vi "Add Service.vi"(6 "WebSocket Data Handler":refnum<class "WebSocket Data Handler Msg.lvclass">, 8 "error in (no error)":errorcluster, 9 "Subscriber Enqueuer":refnum<class "Message Enqueuer.lvclass">, 10 "Service Name":string, 11 "WebSocket Server in":refnum<class "WebSocket Server.lvclass">) -> (0 "error out":errorcluster, 3 "WebSocket Server out":refnum<class "WebSocket Server.lvclass">)   [LabVIEW 2016, in "WebSocket Actor.lvlib" / "WebSocket Server.lvclass"]
uses:
  WebSocket Server.lvclass
  C:/Program Files (x86)/National Instruments/LabVIEW 2016/vi.lib/ActorFramework/Actor/Actor.lvclass
  <vilib>/ActorFramework/Message Enqueuer/Message Enqueuer.lvclass
  Abstract Messages/WebSocket Data Handler Msg/WebSocket Data Handler Msg.lvclass
  WebSocket Server.lvclass/WebSocket Server.ctl
  WebSocket Listener Actor/WebSocket Service Actor.lvclass
  WebSocket Listener Actor/WebSocket Service Actor.lvclass/WebSocket Service Actor.ctl
  Abstract Messages/WebSocket Service Enqueuer Msg/WebSocket Service Enqueuer Msg.lvclass/WebSocket Service Enqueuer Msg.ctl
  <vilib>/ActorFramework/Message Enqueuer/Message Enqueuer.lvclass/Message Enqueuer.ctl
  WebSocket Listener Actor/properties/Write Subscriber Enqueuer.vi
  WebSocket Listener Actor/properties/Write WebSocket Data Handler.vi
  <vilib>/ActorFramework/Message Enqueuer/Enqueue.vi
  Abstract Messages/WebSocket Service Enqueuer Msg/WebSocket Service Enqueuer Msg.lvclass
  C:/Program Files (x86)/National Instruments/LabVIEW 2016/vi.lib/ActorFramework/Message/Message.lvclass
  <vilib>/ActorFramework/Message Priority Queue/Priority Enqueue.vi
  <vilib>/ActorFramework/Actor/Actor.lvclass
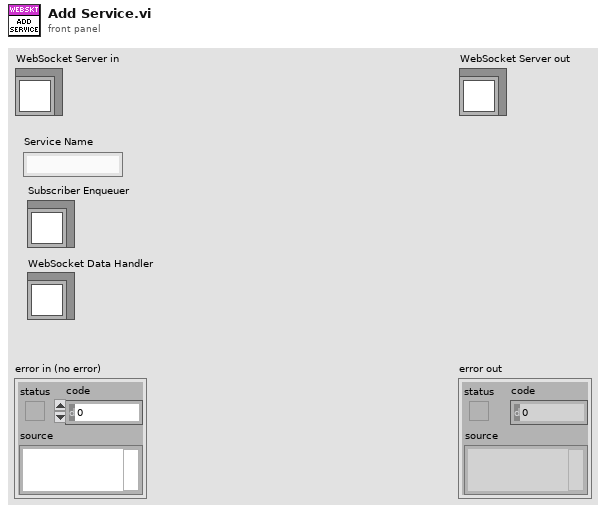
[diagram p1: front panel]
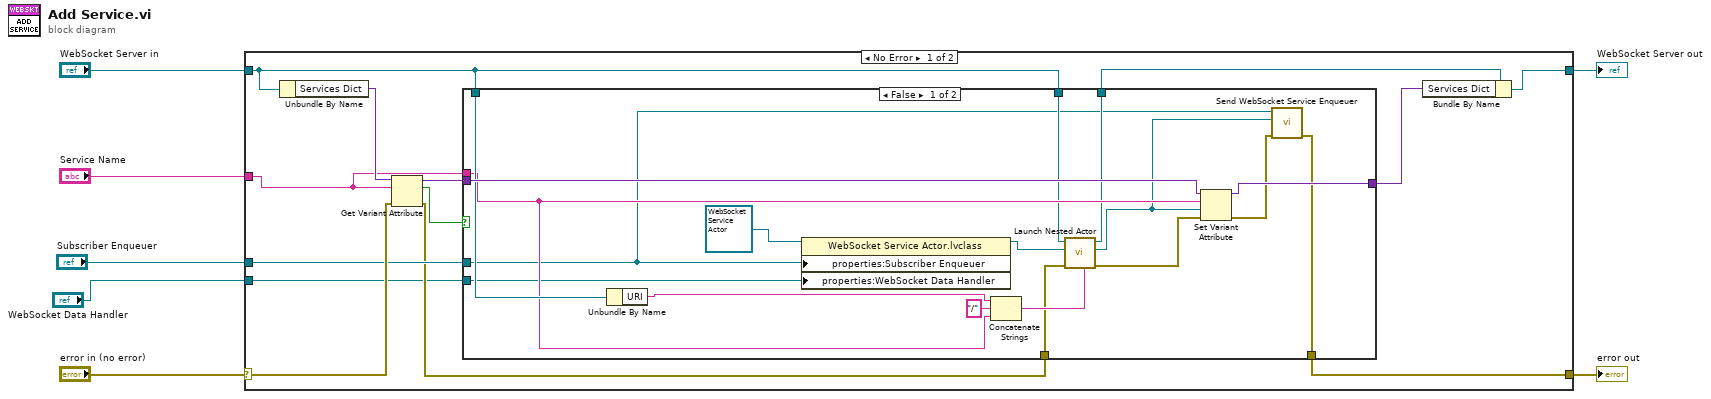
[diagram p0: block diagram]
diagram:
  n1 = case shown="No Error" "error in (no error)" {
    selector: "error in (no error)" -> [w17 w43]
    tunnel: [w14 w43] -> w6
    tunnel: [w20 w42] -> w4
    tunnel: "WebSocket Server in" -> [w9 w42]
    tunnel: "Service Name" -> [w16 _]
    tunnel: "Subscriber Enqueuer" -> [w11 _]
    tunnel: "WebSocket Data Handler" -> [w8 _]
    frame No Error {
      n2 = Unbundle By Name(w9) -> ("Services Dict"=w19:variant)
      n3 = Get Variant Attribute(Variant=w19, name=w16, error in=w17) -> (duplicate Variant=w13:variant, found=w18:bool, error out=w10:errorcluster)  [unwired: 1 in, 1 out]
      n4 = case shown="False" w18 {
        tunnel: w16 -> [w31 _]
        tunnel: [w26 w40] -> w15
        tunnel: [w23 w39] -> w14
        tunnel: w13 -> [w38 w41]
        tunnel: [w37 w41] -> w12
        tunnel: w9 -> [w36 _]
        tunnel: w11 -> [w21 _]
        tunnel: w10 -> [w30 w39]
        tunnel: w9 -> [w27 w40]
        tunnel: w8 -> [w25 _]
        frame False {
          n5 = Unbundle By Name(w36) -> ("URI"=w32:string)
          n6 = property class="WebSocket Service Actor.lvclass"(reference=refnum<class "WebSocket Service Actor.lvclass"> refnum ("WebSocket Actor.lvlib:WebSocket Service Actor.lvclass"), "properties:Subscriber Enqueuer"=w21, "properties:WebSocket Data Handler"=w25) -> (reference out=w28:refnum<class "WebSocket Service Actor.lvclass">)  [unwired: 1 in, 1 out]
          n7 = Concatenate Strings(w32, "/" ("string"), w31) -> (w34:string)
          n8 = call <vilib>:"Launch Nested Actor.vi"("Debug Alias"=w34, "error in (no error)"=w30, "Nested Actor"=w28, "Caller Actor in"=w27) -> ("error out"=w29:errorcluster, "Nested Actor's Enqueuer"=w22:refnum<class "Message Enqueuer.lvclass">, "Caller Actor out"=w26:refnum<class "WebSocket Server.lvclass">)  [unwired: 5 in]
          n9 = Set Variant Attribute(Variant=w38, name=w31, value=w22, error in=w29) -> (Variant out=w37:variant, error out=w24:errorcluster)  [unwired: 1 out]
          n10 = call "Send WebSocket Service Enqueuer.vi"("error in (no error)"=w24, "WebSocket Service Enqueuer"=w22, "Message Enqueuer"=w21) -> ("error out"=w23:errorcluster)  [unwired: 7 in, 1 out]
        }
        frame True {
        }
      }
      n11 = Bundle By Name(cluster=w15, "Services Dict"=w12) -> (w20:refnum<class "WebSocket Server.lvclass">)
    }
    frame Error {
    }
  }
  "error out" <- w6
  "WebSocket Server out" <- w4
